vi "Koheras_Initilisation.vi"(5 "error in":errorcluster) -> (19 "error out":errorcluster)   [LabVIEW 2011]
uses:
  Variables/GlobalGetKoherasLaserOnOff.vi
  Utilities/globalvariables/KoherasGetSetStatus.vi
  Variables/KoherasStatus.vi
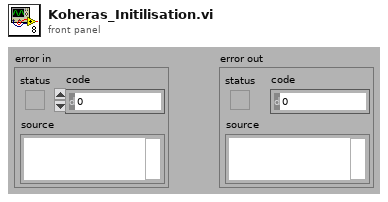
[diagram p1: front panel]
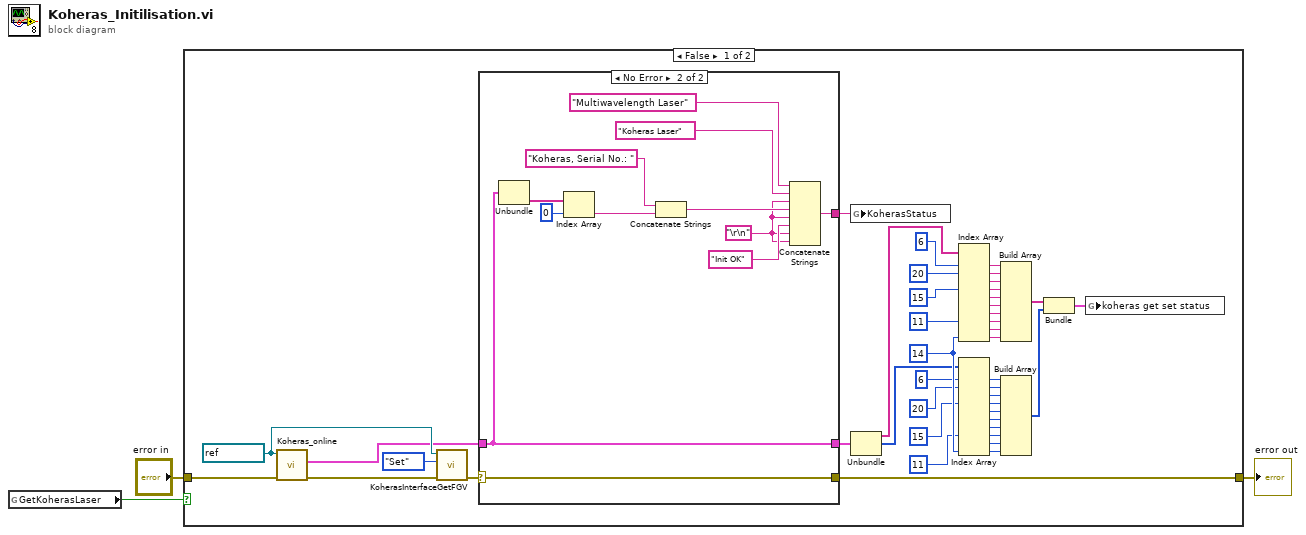
[diagram p0: block diagram]
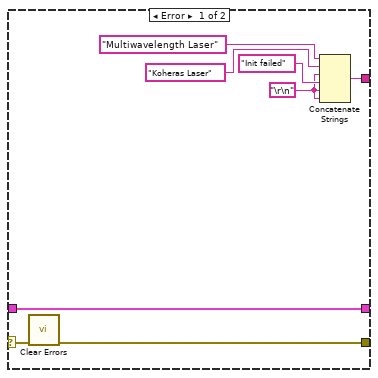
[diagram p2: hidden frame]
diagram:
  n1 = global read "GlobalGetKoherasLaserOnOff.vi" "GetKoherasLaser"() -> (w1:bool)
  n2 = case shown="False" w1 {
    tunnel: [w4 w67] -> w3
    tunnel: "error in" -> [w46 w67]
    frame False {
      w40 = 14 ("index")
      w44 = refnum<visa-resource-name> "COM3" ("VISA resource name")
      n3 = call "Koheras_online.vi"("error in"=w46, "VISA resource name"=w44) -> ("error out"=w45:errorcluster, "Result"=w8:cluster{string[], i32[], "Return":string[]})  [unwired: 7 in, 1 out]
      n4 = call "KoherasInterfaceGetFGV.vi"(8:"in"=w45, "Set_Get"=enum16{"Set", "Get"}."Set", 11:"in"=w44) -> ("out"=w7:errorcluster)  [unwired: 7 in, 1 out]
      n5 = case shown="No Error" w7 {
        selector: w7 -> [w48 w56]
        tunnel: [w52 w65] -> w6
        tunnel: [w51 w56] -> w4
        tunnel: w8 -> [w49 w57]
        tunnel: [w49 w57] -> w41
        frame Error {
          w50 = "\r\n"
          n6 = call <vilib>:"Clear Errors.vi"("error in (no error)"=w48) -> ("error out"=w51:errorcluster)  [unwired: 6 in]
          n7 = Concatenate Strings("Multiwavelength Laser" ("string"), "Koheras Laser" ("string"), w50, "Init failed" ("string"), w50, w50) -> (w52:string)
        }
        frame No Error {
          w58 = "\r\n"
          n8 = Unbundle(w57) -> ("Return"=w61:string[])  [unwired: 2 out]
          n9 = Index Array(array=w61, index=0) -> (element=w59:string)
          n10 = Concatenate Strings("Koheras, Serial No.: " ("string"), w59) -> (w63:string)
          n11 = Concatenate Strings("Multiwavelength Laser" ("string"), "Koheras Laser" ("string"), w58, w63, w58, "Init OK" ("string"), w58, w58) -> (w65:string)
        }
      }
      n12 = global write "KoherasStatus.vi" "KoherasStatus"(w6) -> ()
      n13 = Unbundle(w41) -> (w10:string[], w13:i32[])  [unwired: 1 out]
      n14 = Index Array(array=w10, index #1=6 ("index"), index #2=20 ("index"), index #4=15 ("index"), index #8=11 ("index"), index #10=w40) -> (element #1=w14:string, element #2=w18:string, element #3=w19:string, element #4=w23:string, element #5=w26:string, element #6=w27:string, element #7=w28:string, element #8=w34:string, element #9=w35:string, element #10=w36:string)  [unwired: 5 in]
      n15 = Index Array(array=w13, index #1=6 ("index"), index #2=20 ("index"), index #4=15 ("index"), index #8=11 ("index"), index #10=w40) -> (element #1=w15:i32, element #2=w20:i32, element #3=w21:i32, element #4=w22:i32, element #5=w29:i32, element #6=w30:i32, element #7=w31:i32, element #8=w37:i32, element #9=w38:i32, element #10=w39:i32)  [unwired: 5 in]
      n16 = Build Array(w14, w18, w19, w23, w26, w27, w28, w34, w35, w36) -> (w42:string[])
      n17 = Build Array(w15, w20, w21, w22, w29, w30, w31, w37, w38, w39) -> (w43:i32[])
      n18 = Bundle(w42, w43) -> (w5:cluster{string[], i32[]})  [unwired: 1 in]
      n19 = global write "KoherasGetSetStatus.vi" "koheras get set status"(w5) -> ()
    }
    frame True {
    }
  }
  "error out" <- w3
